vi "InitializeWheelSpinnerSystem.vi"   [LabVIEW 2019]
uses:
  <vilib>/Rock Robotics/WPI/Solenoid/WPI_SolenoidOpenSingle.vi
  <vilib>/Rock Robotics/WPI/Solenoid/WPI_SolenoidChannel.ctl
  <vilib>/Rock Robotics/SystemInterfaces/i2clib/i2c_bus.ctl
  <vilib>/Rock Robotics/SystemInterfaces/DIO/FPGA_DIOPWMChannel.ctl
  <vilib>/Rock Robotics/WPI/MotorControl/WPI_MotorControlOpen VictorSPX.vi
types:
  T1 = typedef "FPGA_DIOPWMChannel.ctl" = enum8{"PWM 0", "PWM 1", "PWM 2", "PWM 3", "PWM 4", "PWM 5", "PWM 6", "PWM 7", "PWM 8", "PWM 9", "PWM MXP 0", "PWM MXP 1", "PWM MXP 2", "PWM MXP 3", "PWM MXP 4", "PWM MXP 5", "PWM MXP 6", "PWM MXP 7", "PWM MXP 8", "PWM MXP 9", "Invalid"}
  T2 = typedef "i2c_bus.ctl" = enum16{"I2C On-Board", "I2C MXP", "Invalid"}
  T3 = typedef "WPI_SolenoidChannel.ctl" = enum8{"Solenoid 0", "Solenoid 1", "Solenoid 2", "Solenoid 3", "Solenoid 4", "Solenoid 5", "Solenoid 6", "Solenoid 7", "Invalid"}
  T4 = typedef "WPI_SolenoidDevRef.ctl" = cluster{"DevStatus":errorcluster, "Pneumatics Control Module":u8, "Forward Solenoid Channel":T3, "Reverse Solenoid Channel":T3}
  T5 = typedef "Color Sensor V3 DevRef.ctl" = cluster{"I2CDevRef":T6}
  T6 = typedef "WPI_I2CDevRef.ctl" = cluster{"DevStatus":errorcluster, "Device Address":u8, "Handle":i32, "I2C Bus":T2}
  T7 = typedef "WPI_MotorControlDeviceRef.ctl" = cluster{"DeviceStatus":errorcluster, "Type":T8, "PWM":cluster{"PWM Channel":T1, "DeadBand":T9}, "CAN":cluster{"Device Number":u8, "SetOutput VI Ref":variant, "GetOutput VI Ref":variant, "Enable VI Ref":variant, "Disable VI Ref":variant, "Data":variant}, "Invert":bool, "DIO PWM":cluster{"PWM \"Enable\" Channel":T1, "DIOChannel":T10, "PWM Rate":dbl}}
  T8 = typedef "WPI_MotorControlType.ctl" = enum16{"PWM", "CAN", "DIO PWM"}
  T9 = typedef "WPI_PWMDeadband.ctl" = cluster{"Name":string, "maxPositivePwm":i32, "minPositivePwm":i32, "centerPwm":i32, "maxNegativePwm":i32, "minNegativePwm":i32, "angularRange":u16}
  T10 = typedef "FPGA_DIOChannel.ctl" = enum8{"DIO 0", "DIO 1", "DIO 2", "DIO 3", "DIO 4", "DIO 5", "DIO 6", "DIO 7", "DIO 8", "DIO 9", "DIO MXP 0", "DIO MXP 1", "DIO MXP 2", "DIO MXP 3", "DIO MXP 4", "DIO MXP 5", "DIO MXP 6", "DIO MXP 7", "DIO MXP 8", "DIO MXP 9", "DIO MXP 10", "DIO MXP 11", "DIO MXP 12", "DIO MXP 13", "DIO MXP 14", "DIO MXP 15", "SPI Port CS1", "SPI Port CS2", "SPI Port CS3", "SPI Port MISO", "SPI Port MOSI", "Invalid"}
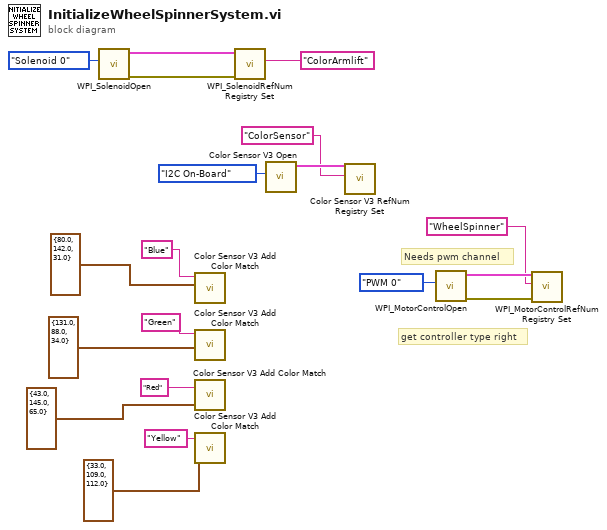
[diagram p0: block diagram]
diagram:
  # "get controller type right"
  # "Needs pwm channel"
  n1 = call-poly <vilib>:"WPI_SolenoidOpen.vi"("Solenoid Channel"=WPI_SolenoidChannel."Solenoid 0") -> ("error out"=w16:errorcluster, "SolenoidDevRef"=w17:T4)  [unwired: 9 in]
  n2 = call <vilib>:"Color Sensor V3 Add Color Match.vi"("Color"=cluster{"R":dbl, "B":dbl, "G":dbl} {"R"=80.0, "B"=142.0, "G"=31.0}, "Name"="Blue") -> ()  [unwired: 10 in]
  n3 = call <vilib>:"Color Sensor V3 Add Color Match.vi"("Color"=cluster{"R":dbl, "G":dbl, "B":dbl} {"R"=131.0, "G"=88.0, "B"=34.0}, "Name"="Green") -> ()  [unwired: 10 in]
  n4 = call <vilib>:"Color Sensor V3 Add Color Match.vi"("Color"=cluster{"R":dbl, "G":dbl, "B":dbl} {"R"=43.0, "G"=145.0, "B"=65.0}, "Name"="Red") -> ()  [unwired: 10 in]
  n5 = call <vilib>:"Color Sensor V3 Add Color Match.vi"("Color"=cluster{"R":dbl, "G":dbl, "B":dbl} {"R"=33.0, "G"=109.0, "B"=112.0}, "Name"="Yellow") -> ()  [unwired: 10 in]
  n6 = call <vilib>:"WPI_SolenoidRefNum Registry Set.vi"("error in (no error)"=w16, "refnum name"="ColorArmlift", "SolenoidDevRef"=w17) -> ()  [unwired: 7 in, 2 out]
  n7 = call <vilib>:"Color Sensor V3 Open.vi"("I2C Bus"=i2c_bus."I2C On-Board") -> ("ColorSensorDevRef"=w15:T5)  [unwired: 9 in, 1 out]
  n8 = call <vilib>:"Color Sensor V3 RefNum Registry Set.vi"("refnum name"="ColorSensor", "ColorSensorDevRef"=w15) -> ()  [unwired: 8 in, 2 out]
  n9 = call-poly <vilib>:"WPI_MotorControlOpen.vi"("PWM Channel"=FPGA_DIOPWMChannel."PWM 0") -> ("error out"=w7:errorcluster, "MotorControlDeviceRef"=w8:T7)  [unwired: 9 in]
  n10 = call <vilib>:"WPI_MotorControlRefNum Registry Set.vi"("error in (no error)"=w7, "refnum name"="WheelSpinner", "MotorControlDevRef"=w8) -> ()  [unwired: 7 in, 2 out]
